vi "Append to Data (Dictionary).vi"(8 "error in (no error)":errorcluster, 10 "key-value":cluster{"key":string, "value":variant}, 11 "Data Save":refnum<class "Data.lvclass">) -> (0 "error out":errorcluster, 3 "Data Save out":refnum<class "Data.lvclass">)   [LabVIEW 2019, in "Data.lvclass"]
uses:
  Data.lvclass
  Typedefs/Dictionary--cluster.ctl
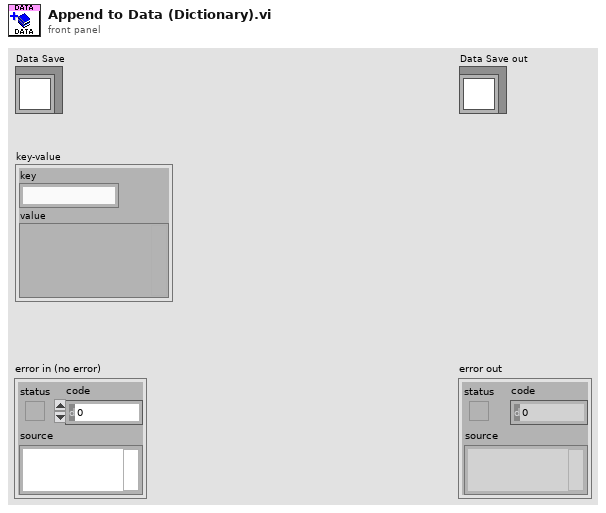
[diagram p1: front panel]
types:
  T1 = typedef "Data.lvclass/Dictionary--cluster.ctl" = cluster{"key":string, "value":variant}
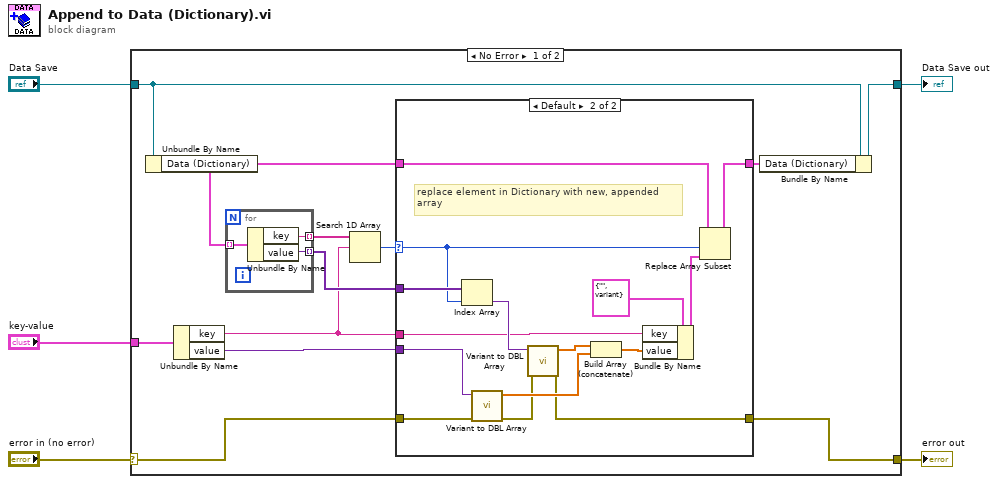
[diagram p0: block diagram]
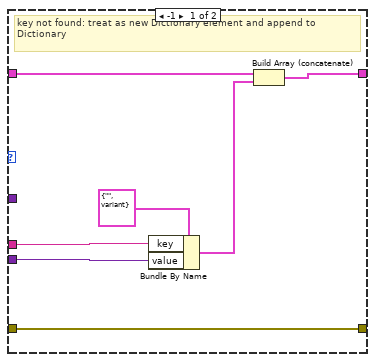
[diagram p2: hidden frame]
diagram:
  n1 = case shown="No Error" "error in (no error)" {
    selector: "error in (no error)" -> [w10 w43]
    tunnel: [w9 w43] -> w4
    tunnel: [w17 w44] -> w2
    tunnel: "Data Save" -> [w16 w44]
    tunnel: "key-value" -> [w14 _]
    frame No Error {
      n2 = Unbundle By Name(w16) -> ("Data (Dictionary)"=w8:T1[])
      n3 = Unbundle By Name(w14) -> ("key"=w12:string, "value"=w11:variant)
      n4 = for {
        tunnel: w8 -> [w40] mode=indexing
        tunnel: [w42] -> w15 mode=indexing
        tunnel: [w41] -> w13 mode=indexing
        n5 = Unbundle By Name(w40) -> ("key"=w42:string, "value"=w41:variant)
      }
      n6 = Search 1D Array(1D array=w15, element=w12) -> (index of element=w6:i32)  [unwired: 1 in]
      n7 = case shown="Default" w6 {
        selector: w6 -> [_ w27]
        tunnel: w13 -> [_ w33]
        tunnel: w12 -> [w24 w32]
        tunnel: w11 -> [w23 w31]
        tunnel: w10 -> [w18 w30]
        tunnel: [w18 w29] -> w9
        tunnel: w8 -> [w21 w26]
        tunnel: [w19 w25] -> w7
        frame -1 {
          # "key not found: treat as new Dictionary element and append to Dictionary"
          n8 = Bundle By Name(cluster=T1 {"key"="", "value"=variant} ("key-value"), "key"=w24, "value"=w23) -> (w20:T1)
          n9 = Build Array (concatenate)(w21, w20) -> (w19:T1[])
        }
        frame Default {
          # "replace element in Dictionary with new, appended\narray"
          n10 = Index Array(array=w33, index=w27) -> (element=w39:variant)
          n11 = call "Variant to DBL Array.vi"("error in (no error)"=w30, "Data (Variant)"=w31) -> ("error out"=w28:errorcluster, "1D Array"=w37:dbl[])  [unwired: 7 in, 1 out]
          n12 = call "Variant to DBL Array.vi"("error in (no error)"=w28, "Data (Variant)"=w39) -> ("error out"=w29:errorcluster, "1D Array"=w38:dbl[])  [unwired: 7 in, 1 out]
          n13 = Build Array (concatenate)(w38, w37) -> (w35:dbl[])
          n14 = Bundle By Name(cluster=T1 {"key"="", "value"=variant} ("key-value"), "key"=w32, "value"=w35) -> (w36:T1)
          n15 = Replace Array Subset(array=w26, new element=w36, index=w27) -> (w25:T1[])
        }
      }
      n16 = Bundle By Name(cluster=w16, "Data (Dictionary)"=w7) -> (w17:refnum<class "Data.lvclass">)
    }
    frame Error {
    }
  }
  "error out" <- w4
  "Data Save out" <- w2
